vi "StartStop.vi"(8 "error in (no error)":errorcluster, 10 "Start? (F)":bool, 11 "VISA resource name":refnum<visa-resource-name>) -> (0 "error out":errorcluster, 3 "VISA resource name out":refnum<visa-resource-name>)   [LabVIEW 2012, in "Surelite I.lvlib"]
doc: "Resets the instrument and then sends a set of default setup commands to the instrument."
uses:
  Surelite I.lvlib
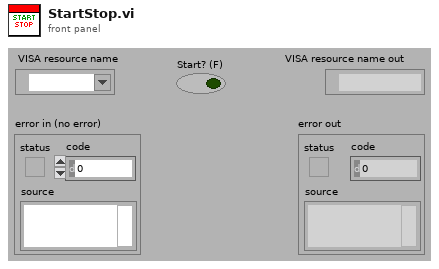
[diagram p1: front panel]
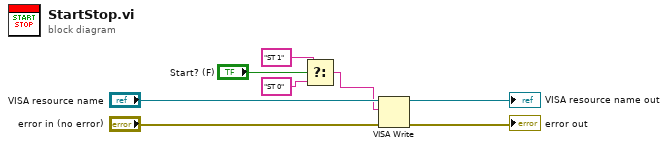
[diagram p0: block diagram]
diagram:
  n1 = Select(t="ST 1", s="Start? (F)", f="ST 0") -> (s? t:f=w4:string)
  n2 = VISA Write(VISA resource name="VISA resource name", write buffer=w4, error in (no error)="error in (no error)") -> (VISA resource name out=→"VISA resource name out":refnum<visa-resource-name>, error out=→"error out":errorcluster)  [unwired: 1 out]
